vi "Create.vi"(8 "error in (no error)":errorcluster, 11 "Motor Controller in":refnum<class "Motor Controller.lvclass">) -> (0 "error out":errorcluster, 3 "Motor Controller out":refnum<class "Motor Controller.lvclass">)   [LabVIEW 2022 SP3, in "Motor Controller.lvclass"]
uses:
  Motor Controller.lvclass
  Motor Controller.lvclass/Motor Controller.ctl
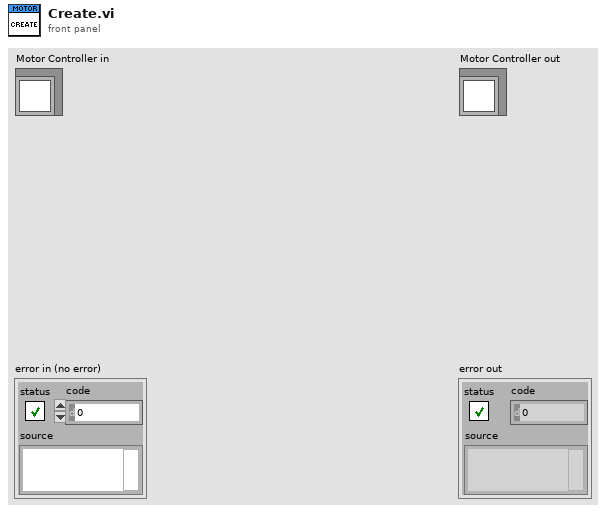
[diagram p1: front panel]
types:
  T1 = typedef "Motor Controller.lvclass/Private Data.ctl" = cluster{"UserEvents":T2, "All Dependencies":cluster{"Class References":refnum<class>[], "Class Names":string[]}, "Status":T3}
  T2 = typedef "Motor Controller.lvclass/UserEvents.ctl" = cluster{"API Incoming Event":refnum<user-event>, "API Executed Event":refnum<user-event>, "API Return Event":refnum<user-event>, "Status Changed Event":refnum<user-event>, "StopEvent":refnum<user-event>}
  T3 = typedef "Motor Controller.lvclass/Status.ctl" = cluster{"Motor Controller Config Data":T4, "Motor Controller Data":cluster{"Enabled?":bool}, "Stage Move":T5, "Stage Busy?":bool}
  T4 = typedef "Motor Controller.lvclass/Motor Controller Config Data.ctl" = cluster{"Motor IP Addresss":string, "Current Position":i32, "Pulse_Per_mm":i32, "PrePrint":dbl[], "Load Position_mm":i32, "Laminate Position_mm":i32}
  T5 = typedef "Motor Controller.lvclass/Stage Move Data.ctl" = cluster{"Current Step":string, "Move Data":T6[]}
  T6 = typedef "Motor Controller.lvclass/Batch Index Speed Data.ctl" = cluster{"Batch & Cycle":string, "Move":cluster{"Index_mm":i32, "Speed_mm_s":i32}, "Status":T7}
  T7 = typedef "Motor Controller.lvclass/Move Status.ctl" = enum16{"Pending", "In Progress", "Completed"}
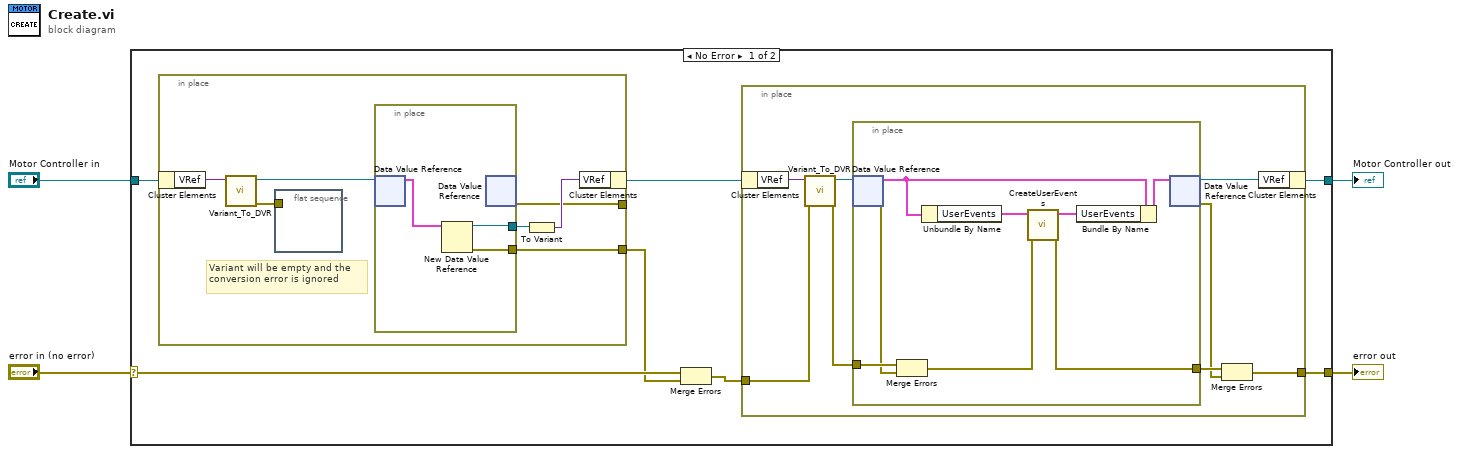
[diagram p0: block diagram]
diagram:
  n1 = case shown="No Error" "error in (no error)" {
    selector: "error in (no error)" -> [w11 w39]
    tunnel: [w5 w39] -> w3
    tunnel: [w7 w38] -> w1
    tunnel: "Motor Controller in" -> [w10 w38]
    frame No Error {
      n2 = in-place {
        in-place-border: [w29] -> _
        in-place-border: [w28] -> w9
        # "Variant will be empty and the conversion error is ignored"
        n3 = in-place-cluster #1(w10) -> ("VRef"=w34:variant)
        n4 = call "Variant_To_DVR.vi"("Variant"=w34) -> ("error out"=w33:errorcluster, "DVR"=w32:refnum<data-value>)  [unwired: 9 in]
        n5 = flat-sequence {
          tunnel: w33 -> [_]
          frame #0 {
          }
        }
        n6 = in-place {
          in-place-border: [w36] -> w31
          in-place-border: [w35] -> w28
          n7 = in-place-dvr #2(w32) -> (w37:T1)  [unwired: 1 out]
          n8 = New Data Value Reference(data value=w37) -> (data value reference=w36:refnum<data-value>, error out=w35:errorcluster)  [unwired: 1 in]
          n9 = in-place-dvr #2() -> (w29:errorcluster)  [unwired: 1 in, 1 out]
        }
        n10 = To Variant(anything=w31) -> (Variant=w30:variant)
        n11 = in-place-cluster #1("VRef"=w30) -> (w8:refnum<class "Motor Controller.lvclass">)
      }
      n12 = Merge Errors(w11, w9) -> (w6:errorcluster)
      n13 = in-place {
        in-place-border: w6 -> [w17]
        in-place-border: [w13] -> w5
        n14 = in-place-cluster #3(w8) -> ("VRef"=w19:variant)
        n15 = call "Variant_To_DVR.vi"("error in (no error)"=w17, "Variant"=w19) -> ("error out"=w16:errorcluster, "DVR"=w18:refnum<data-value>)  [unwired: 8 in]
        n16 = in-place {
          in-place-border: w16 -> [w23]
          in-place-border: [w20] -> w15
          n17 = in-place-dvr #4(w18) -> (w26:T1, w21:errorcluster)
          n18 = Merge Errors(w23, w21) -> (w22:errorcluster)
          n19 = Unbundle By Name(w26) -> ("UserEvents"=w27:T2)
          n20 = call "CreateUserEvents.vi"("error in (no error)"=w22, "UserEvents"=w27) -> ("error out"=w20:errorcluster, "UserEvents out"=w25:T2)  [unwired: 8 in]
          n21 = Bundle By Name(cluster=w26, "UserEvents"=w25) -> (w24:T1)
          n22 = in-place-dvr #4(w24) -> (w12:refnum<data-value>, w14:errorcluster)
        }
        n23 = Merge Errors(w15, w14) -> (w13:errorcluster)
        n24 = in-place-cluster #3("VRef"=w12) -> (w7:refnum<class "Motor Controller.lvclass">)
      }
    }
    frame Error {
    }
  }
  "error out" <- w3
  "Motor Controller out" <- w1
